vi "Configure Frequency (Start Stop).vi"(0 "VISA resource name":refnum<visa-resource-name>, 5 "Start Frequency (0Hz)":dbl min=-100000000.0 max=43100000000.0, 7 "Stop Frequency (3000000000Hz)":dbl=3000000000.0 min=-99997000.0 max=43100000000.0, 11 "error in (no error)":errorcluster) -> (4 "VISA resource name out":refnum<visa-resource-name>, 15 "error out":errorcluster)   [LabVIEW 2023, in "Anritsu Signal Analyzer Series.lvlib"]
doc: "Configures the frequency range defining its start frequency and its stop frequency."
uses:
  Anritsu Signal Analyzer Series.lvlib
panel:
  # "Hz"
  # "Hz"
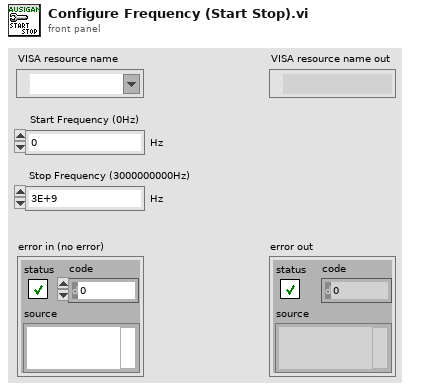
[diagram p1: front panel]
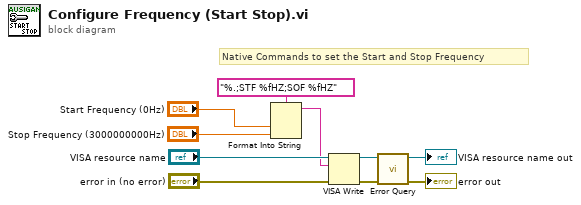
[diagram p0: block diagram]
diagram:
  # "Native Commands to set the Start and Stop Frequency"
  n1 = Format Into String(format string="%.;STF %fHZ;SOF %fHZ" ("Format String"), "Start Frequency (0Hz)", "Stop Frequency (3000000000Hz)") -> (resulting string=w1:string)  [unwired: 2 in, 1 out]
  n2 = VISA Write(VISA resource name="VISA resource name", write buffer=w1, error in (no error)="error in (no error)") -> (VISA resource name out=w2:refnum<visa-resource-name>, error out=w3:errorcluster)  [unwired: 1 out]
  n3 = call "Error Query.vi"("error in (no error)"=w3, "VISA resource name"=w2) -> ("error out"=→"error out":errorcluster, "VISA resource name out"=→"VISA resource name out":refnum<visa-resource-name>)  [unwired: 6 in, 2 out]
